vi "freedrive.vi"(2 "Input":T2, 3 "Reference":T1) -> (1 "String":string)   [LabVIEW 2024]
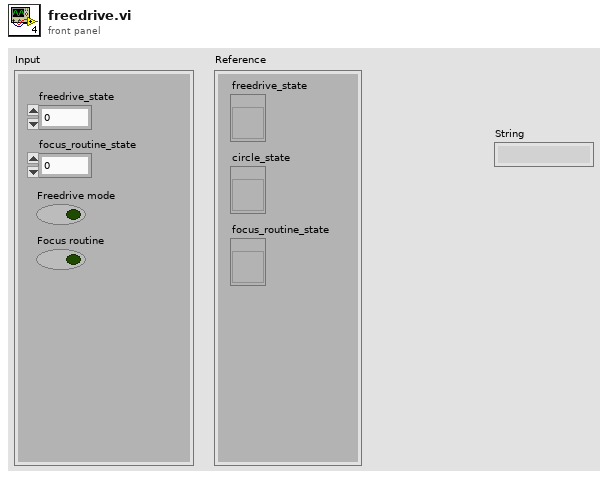
[diagram p1: front panel]
types:
  T1 = cluster{"freedrive_state":refnum<vi>, "circle_state":refnum<vi>, "focus_routine_state":refnum<vi>}
  T2 = cluster{"freedrive_state":i8, "focus_routine_state":i8, "Freedrive mode":bool, "Focus routine":bool}
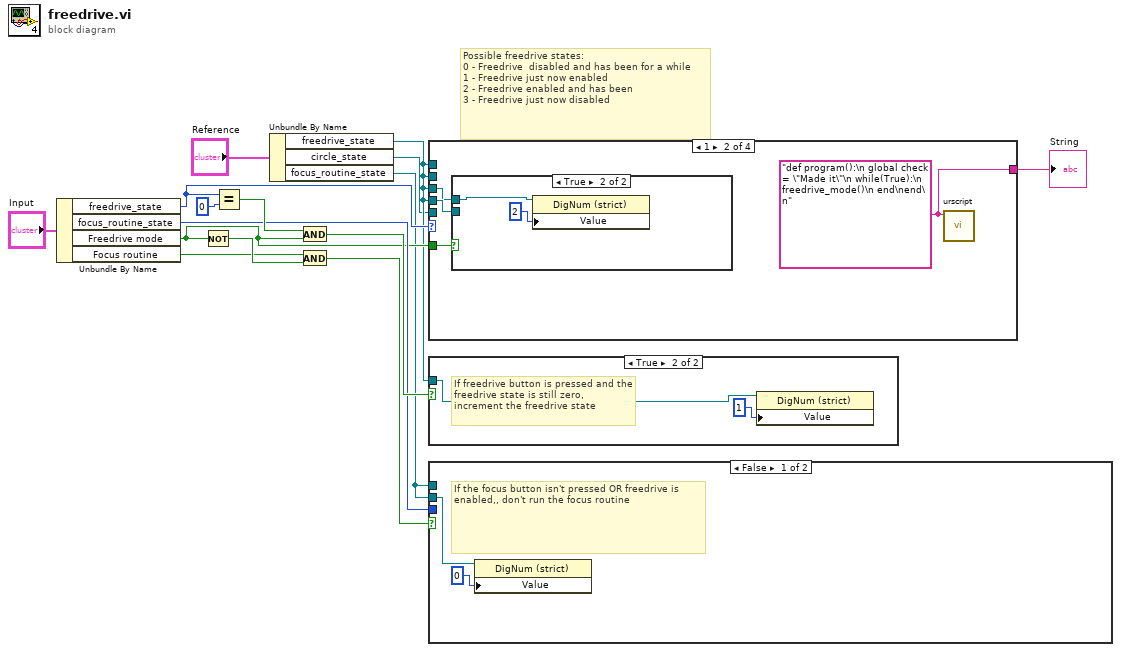
[diagram p0: block diagram]
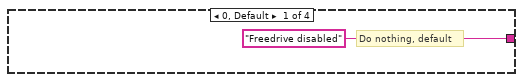
[diagram p3: hidden frame]
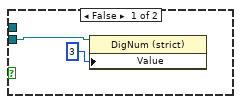
[diagram p4: hidden frame]
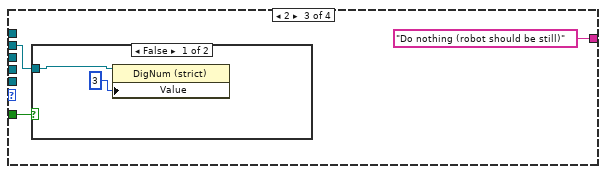
[diagram p5: hidden frame]
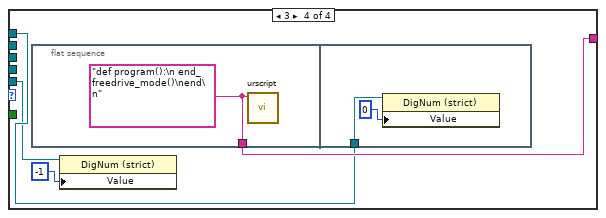
[diagram p7: hidden frame]
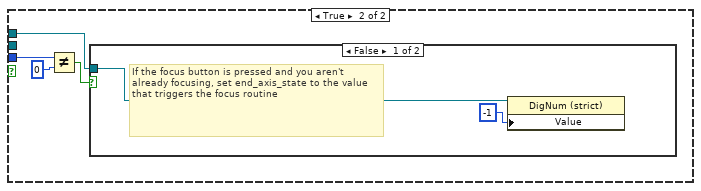
[diagram p8: hidden frame]
diagram:
  # "Possible freedrive states:\n0 - Freedrive  disabled and has been for a while\n1 - Freedrive just now enabled\n2 - Freedrive enabled and has been\n3 - Freedrive just now disabled"
  n1 = Unbundle By Name("Input") -> ("freedrive_state"=w8:i8, "focus_routine_state"=w7:i8, "Freedrive mode"=w6:bool, "Focus routine"=w5:bool)
  n2 = Not(x=w6) -> (.not. x?=w11:bool)
  n3 = Equal?(x=w8, y=0) -> (x = y?=w14:bool)
  n4 = Unbundle By Name("Reference") -> ("freedrive_state"=w3:refnum<vi>, "circle_state"=w2:refnum<vi>, "focus_routine_state"=w1:refnum<vi>)
  n5 = And(x=w14, y=w6) -> (x .and. y?=w15:bool)
  n6 = And(x=w5, y=w11) -> (x .and. y?=w10:bool)
  n7 = case shown="1" w8 {
    tunnel: ["Freedrive disabled" w17 "Do nothing (robot should be still)" w33] -> w12
    tunnel: w6 -> [_ w20 w26 _]
    tunnel: w3 -> [_ w19 _ _]
    tunnel: w3 -> [_ w18 _ _]
    tunnel: w3 -> [_ _ w25 _]
    tunnel: w3 -> [_ _ _ w31]
    tunnel: w2 -> [_ _ _ w30]
    frame 0, Default {
      # "Do nothing, default"
    }
    frame 1 {
      w17 = "def program():\n global check = \"Made it\"\n while(True):\n  freedrive_mode()\n end\nend\n"
      n8 = case shown="True" w20 {
        tunnel: w19 -> [w21 _]
        tunnel: w18 -> [_ w23]
        frame False {
          n9 = property class="DigNum (strict)"(reference=w21, "Value"=3) -> ()  [unwired: 1 in, 2 out]
        }
        frame True {
          n10 = property class="DigNum (strict)"(reference=w23, "Value"=2) -> ()  [unwired: 1 in, 2 out]
        }
      }
      n11 = call "urscript.vi"("String"=w17) -> ()  [unwired: 11 in]
    }
    frame 2 {
      n12 = case shown="False" w26 {
        tunnel: w25 -> [w28 _]
        frame False {
          n13 = property class="DigNum (strict)"(reference=w28, "Value"=3) -> ()  [unwired: 1 in, 2 out]
        }
        frame True {
        }
      }
    }
    frame 3 {
      n14 = flat-sequence {
        tunnel: [w34] -> w33
        tunnel: w31 -> [w35]
        frame #0 {
          w34 = "def program():\n end_freedrive_mode()\nend\n"
          n15 = call "urscript.vi"("String"=w34) -> ()  [unwired: 11 in]
        }
        frame #1 {
          n16 = property class="DigNum (strict)"(reference=w35, "Value"=0) -> ()  [unwired: 1 in, 2 out]
        }
      }
      n17 = property class="DigNum (strict)"(reference=w30, "Value"=-1) -> ()  [unwired: 1 in, 2 out]
    }
  }
  "String" <- w12
  n18 = case shown="True" w15 {
    tunnel: w3 -> [_ w37]
    frame False {
    }
    frame True {
      # "If freedrive button is pressed and the freedrive state is still zero, increment the freedrive state"
      n19 = property class="DigNum (strict)"(reference=w37, "Value"=1) -> ()  [unwired: 1 in, 2 out]
    }
  }
  n20 = case shown="False" w10 {
    tunnel: w7 -> [_ w44]
    tunnel: w1 -> [w39 _]
    tunnel: w1 -> [_ w41]
    frame False {
      # "If the focus button isn't pressed OR freedrive is enabled,, don't run the focus routine"
      n21 = property class="DigNum (strict)"(reference=w39, "Value"=0) -> ()  [unwired: 1 in, 2 out]
    }
    frame True {
      n22 = Not Equal?(x=w44, y=0) -> (x != y?=w42:bool)
      n23 = case shown="False" w42 {
        tunnel: w41 -> [w45 _]
        frame False {
          # "If the focus button is pressed and you aren't already focusing, set end_axis_state to the value that triggers the focus routine"
          n24 = property class="DigNum (strict)"(reference=w45, "Value"=-1) -> ()  [unwired: 1 in, 2 out]
        }
        frame True {
          # "If the focus button is pressed but you're already focusing, do nothing"
        }
      }
    }
  }
